vi "sel_obj.vi"(3 "error in":errorcluster, 4 "Object":string="Безымянный" caption="Объект", 5 "DevNo":u32, 6 "conn ref in":T1) -> (0 "error out":errorcluster, 1 "conn ref out":T1, 2 "Obj Id":i32)   [LabVIEW 2010]
uses:
  <vilib>/addons/database/Connection.llb/Conn ObjectReference.ctl
  <vilib>/addons/database/_DB Variant To Data/Database Variant To Data.xnode
  <vilib>/addons/database/NI_Database_API.lvlib
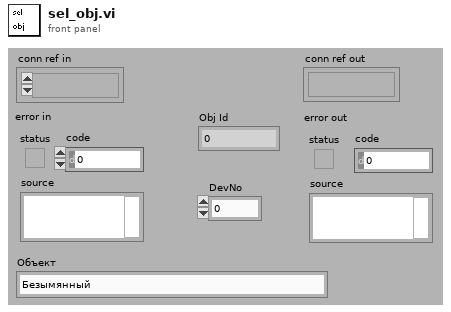
[diagram p1: front panel]
types:
  T1 = typedef "NI_Database_API.lvlib/Conn ObjectReference.ctl" = refnum<k1>
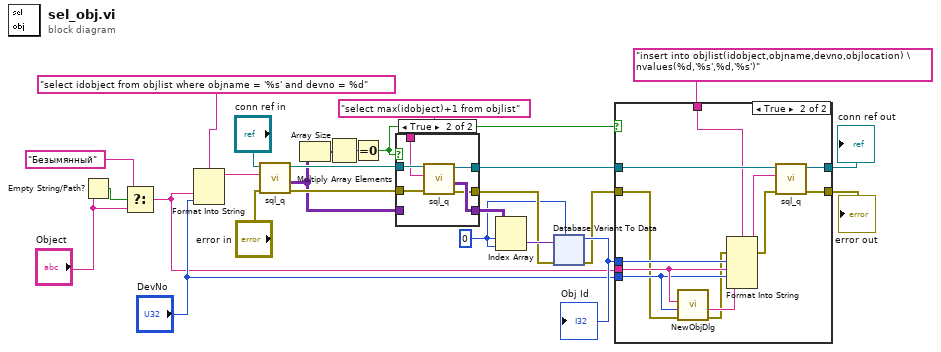
[diagram p0: block diagram]
diagram:
  w6 = 0 ("index (row)")
  n1 = Empty String/Path?(string/path="Object") -> (empty?=w5:bool)
  n2 = Select(t="Безымянный", s=w5, f="Object") -> (s? t:f=w3:string)
  n3 = Format Into String(format string="select idobject from objlist where objname = '%s' and devno = %d" ("table"), w3, "DevNo") -> (resulting string=w18:string)  [unwired: 2 in, 1 out]
  n4 = call "sql_q.vi"("error in"="error in", "SQL query"=w18, "connect ref"="conn ref in") -> ("error out"=w21:errorcluster, "recordset data"=w12:variant[][], "conn ref out"=w22:T1)  [unwired: 1 in, 1 out]
  n5 = Array Size(array=w12) -> (size(s)=w26:i32[])
  n6 = Multiply Array Elements(1:w26) -> (0:w25:i32)
  n7 = Equal To 0?(x=w25) -> (x = 0?=w11:bool)
  n8 = case shown="True" w11 {
    tunnel: w22 -> [w29 w35]
    tunnel: w21 -> [w28 w34]
    tunnel: "select max(idobject)+1 from objlist" ("table") -> [_ w33]
    tunnel: [w27 w32] -> w15
    tunnel: [w29 w31] -> w13
    tunnel: [w28 w30] -> w8
    tunnel: w12 -> [w27 _]
    frame False {
    }
    frame True {
      n9 = call "sql_q.vi"("error in"=w34, "SQL query"=w33, "connect ref"=w35) -> ("error out"=w30:errorcluster, "recordset data"=w32:variant[][], "conn ref out"=w31:T1)  [unwired: 1 in, 1 out]
    }
  }
  n10 = Index Array(array=w15, index (row)=w6, index (col)=w6) -> (element=w14:variant)
  n11 = xnode "Database Variant To Data"("database variant"=w14, "error in"=w8, "type"=w6) -> ("data"=w9:i32, "error out"=w1:errorcluster)
  "Obj Id" <- w9
  n12 = case shown="True" w11 {
    tunnel: [w37 w49] -> w17
    tunnel: [w36 w48] -> w16
    tunnel: w13 -> [w37 w47]
    tunnel: w1 -> [w36 w40]
    tunnel: "insert into objlist(idobject,objname,devno,objlocation) \nvalues(%d,'%s',%d,'%s')" ("table") -> [_ w45]
    tunnel: w3 -> [_ w42]
    tunnel: "DevNo" -> [_ w41]
    tunnel: w9 -> [_ w44]
    frame False {
    }
    frame True {
      n13 = call "NewObjDlg.vi"("error in (no error)"=w40, "DevNo"=w41, "ObjName"=w42) -> ("error out"=w39:errorcluster, "ObjLocation"=w43:string)  [unwired: 2 in, 1 out]
      n14 = Format Into String(format string=w45, error in=w39, w44, w42, w41, w43) -> (resulting string=w46:string, error out=w38:errorcluster)  [unwired: 1 in]
      n15 = call "sql_q.vi"("error in"=w38, "SQL query"=w46, "connect ref"=w47) -> ("error out"=w48:errorcluster, "conn ref out"=w49:T1)  [unwired: 1 in, 2 out]
    }
  }
  "error out" <- w16
  "conn ref out" <- w17
